vi "Append to Array - Null.vi"(8 "error in (no error)":errorcluster, 11 "JSON Tree in (JSON Array)":variant) -> (0 "error out":errorcluster, 3 "JSON Tree out (JSON Array)":variant)   [LabVIEW 2013, in "i3-json.lvlib"]
doc: "Use this template to build a VI to use as a subVI."
uses:
  i3-json.lvlib
  JSON Types/JSON Type.ctl
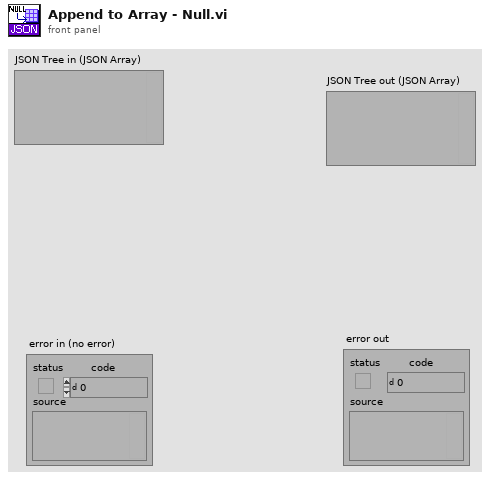
[diagram p1: front panel]
types:
  T1 = typedef "i3-json.lvlib/JSON Type.ctl" = enum8{"JSON Compatible", "JSON Array", "JSON Object", "JSON Null", "Double", "String", "Boolean", "Unknown", "Data JSON string"}
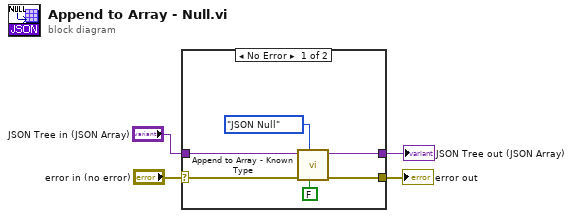
[diagram p0: block diagram]
diagram:
  n1 = case shown="No Error" "error in (no error)" {
    selector: "error in (no error)" -> [w8 w12]
    tunnel: [w9 w12] -> w3
    tunnel: [w10 w11] -> w2
    tunnel: "JSON Tree in (JSON Array)" -> [w7 w11]
    frame No Error {
      n2 = call "Append to Array - Known Type.vi"("Add Parameter as JSON Tree?"=FALSE, "JSON Type"=JSON_Type."JSON Null", "error in (no error)"=w8, "JSON Tree in (JSON Array)"=w7) -> ("error out"=w9:errorcluster, "JSON Tree out (JSON Array)"=w10:variant)  [unwired: 6 in]
    }
    frame Error {
    }
  }
  "error out" <- w3
  "JSON Tree out (JSON Array)" <- w2
